vi "GetNodeMenuOptions.vi"(0 "reference":refnum<class "PackageNode.lvclass">, 1 "MousePos":T1 {"y" format="%.2f"; "x" format="%.2f"}, 5 "error in (no error)":errorcluster) -> (14 "reference out":refnum<class "PackageNode.lvclass">, 15 "MenuOptions":string[](array[string]), 19 "error out":errorcluster)   [LabVIEW 2014, in "PackageNode.lvclass"]
doc: "Gets the menu option"
uses:
  <resource>/Framework/Providers/Open_GDS/UML/PackageNode_class/PackageNode.lvclass
  <resource>/Framework/Providers/Open_GDS/UML/General/Point/Point Point2D.ctl
  <resource>/Framework/Providers/Open_GDS/UML/RectangularNode_class/RectangularNode.lvclass
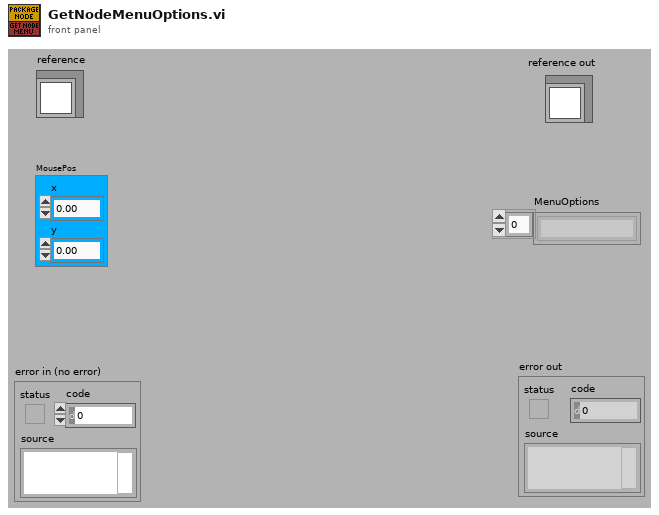
[diagram p1: front panel]
types:
  T1 = typedef "Point Point2D.ctl" = cluster{"x":dbl, "y":dbl}
  T2 = typedef "PackageNode.lvclass/ObjectAttributes.ctl" = cluster{"name":string, "contents":refnum<class "MultiLineString.lvclass">, "DEFAULT_TOP_WIDTH":i32, "DEFAULT_TOP_HEIGHT":i32, "DEFAULT_WIDTH":i32, "DEFAULT_HEIGHT":i32, "NAME_GAP":i32, "XGAP":i32, "YGAP":i32, "Collapsed":bool, "Note color":u32, "Justification":u16}
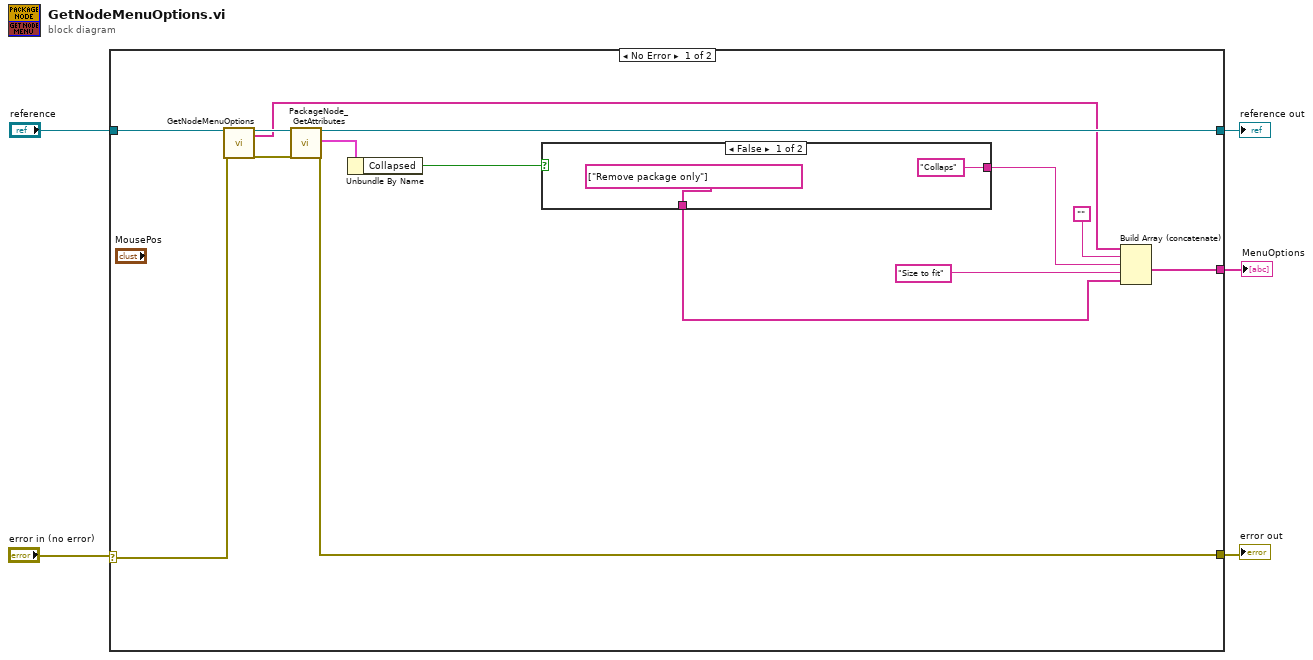
[diagram p0: block diagram]
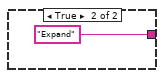
[diagram p2: hidden frame]
diagram:
  n1 = case shown="No Error" "error in (no error)" {
    selector: "error in (no error)" -> [w13 w23]
    tunnel: "reference" -> [w14 w24]
    tunnel: [w19 w23] -> w4
    tunnel: [w18 w24] -> w3
    tunnel: [w17 _] -> w1
    frame No Error {
      n2 = call-parent "GetNodeMenuOptions.vi"("reference"=w14, "error in (no error)"=w13) -> ("reference out"=w15:refnum<class "PackageNode.lvclass">, "MenuOptions"=w10:string[], "error out"=w12:errorcluster)  [unwired: 15 in]
      n3 = call <resource>:"PackageNode_GetAttributes.vi"("reference in"=w15, "error in (no error)"=w12) -> ("reference out"=w18:refnum<class "PackageNode.lvclass">, "Data"=w6:T2, "error out"=w19:errorcluster)  [unwired: 14 in, 1 out]
      n4 = Unbundle By Name(w6) -> ("Collapsed"=w16:bool)
      n5 = case shown="False" w16 {
        tunnel: ["Collaps" "Expand"] -> w8
        tunnel: [string[] ["Remove package only"] _] -> w7
        frame False {
        }
        frame True {
        }
      }
      n6 = Build Array (concatenate)(w10, "", w8, "Size to fit", w7) -> (w17:string[])
    }
    frame Error {
    }
  }
  "reference out" <- w3
  "error out" <- w4
  "MenuOptions" <- w1
